vi "directory exists.vi"(8 "error in":errorcluster, 11 "directory":path) -> (0 "error out":errorcluster, 2 "directory present?":bool, 3 "directory out":path)   [LabVIEW 2013]
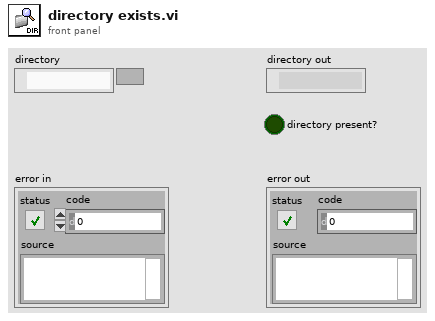
[diagram p1: front panel]
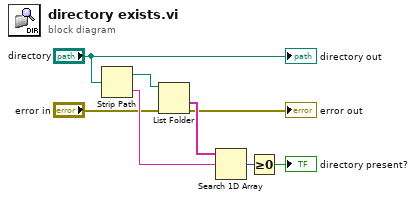
[diagram p0: block diagram]
diagram:
  n1 = Strip Path(path="directory") -> (stripped path=w6:path, name=w4:string)
  n2 = List Folder(path=w6, error in="error in") -> (folder names=w5:string[], error out=→"error out":errorcluster)  [unwired: 2 in, 2 out]
  n3 = Search 1D Array(1D array=w5, element=w4) -> (index of element=w7:i32)  [unwired: 1 in]
  n4 = Greater Or Equal To 0?(x=w7) -> (x >= 0?=→"directory present?":bool)
  "directory out" <- "directory"
